vi "CSMOMgr-Get CSMO.vi"(6 "GenError?(T)":bool=TRUE, 8 "Error in":errorcluster caption="Error in (no error)", 10 "Queue Name":string, 11 "CSMOMgr":T3) -> (0 "Error out":errorcluster, 1 "values":T1={"Requested Name"="", "Module Name"="", "Mode"=enum."Stand Alone", "Queue"=refnum, "CSM-Data"=refnum, "User Event"=refnum, "Status Change Event"=refnum, "Allowed Messages"=[], "Mode-Data"=refnum, "Group Name"="", "Exit Event"=refnum}, 2 "found":bool, 3 "CSMOMgr out":T3)   [LabVIEW 2020, in "Communicable State Machine.lvlib"]
uses:
  Communicable State Machine.lvlib
  Def-CSMOMgr.ctl
  _CSMObj.ctl
  Priority Queue.lvclass
  _CSM_MODE.ctl
  _CSMObj-Data.ctl
  _CSM Status Change Event Data.ctl
  _CSMObj-ModeData.ctl
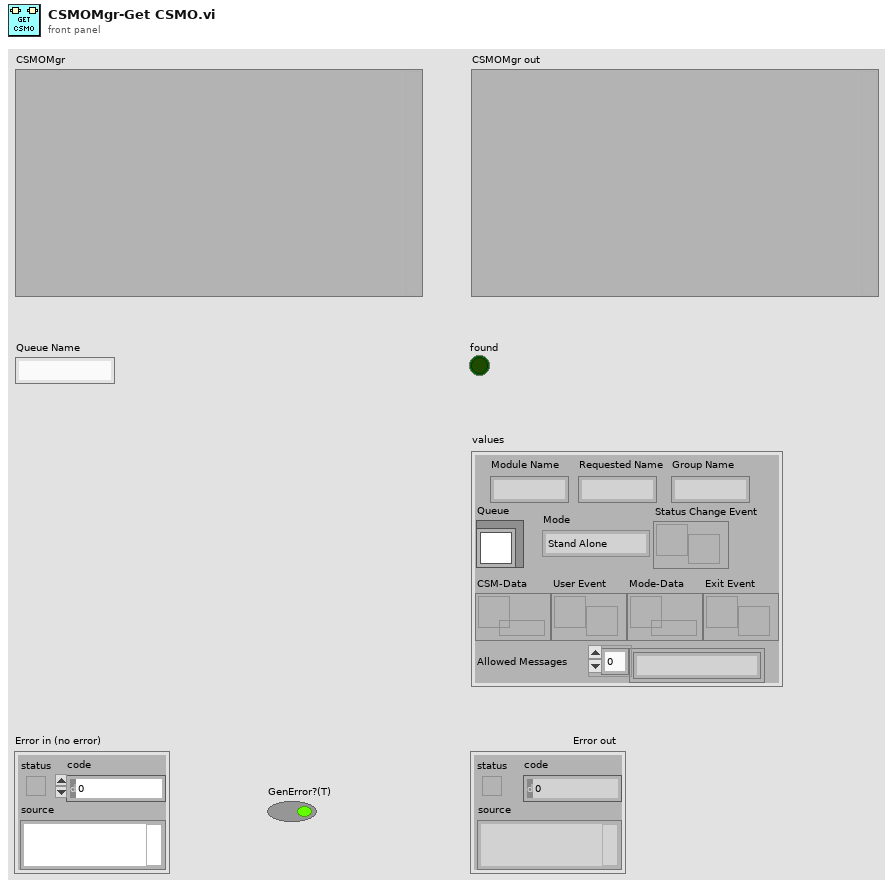
[diagram p1: front panel]
types:
  T1 = typedef "Communicable State Machine.lvlib/_CSMObj.ctl" = cluster{"Requested Name":string, "Module Name":string, "Mode":T2, "Queue":refnum<class "Priority Queue.lvclass">, "CSM-Data":refnum<data-value>, "User Event":refnum<user-event>, "Status Change Event":refnum<user-event>, "Allowed Messages":string[], "Mode-Data":refnum<data-value>, "Group Name":string, "Exit Event":refnum<user-event>}
  T2 = typedef "Communicable State Machine.lvlib/_CSM_MODE.ctl" = enum16{"Not Exist", "Stand Alone", "CSM", "Worker Agent", "Worker", "Chain", "Chain Node"}
  T3 = typedef "Communicable State Machine.lvlib/Def-CSMOMgr.ctl" = variant
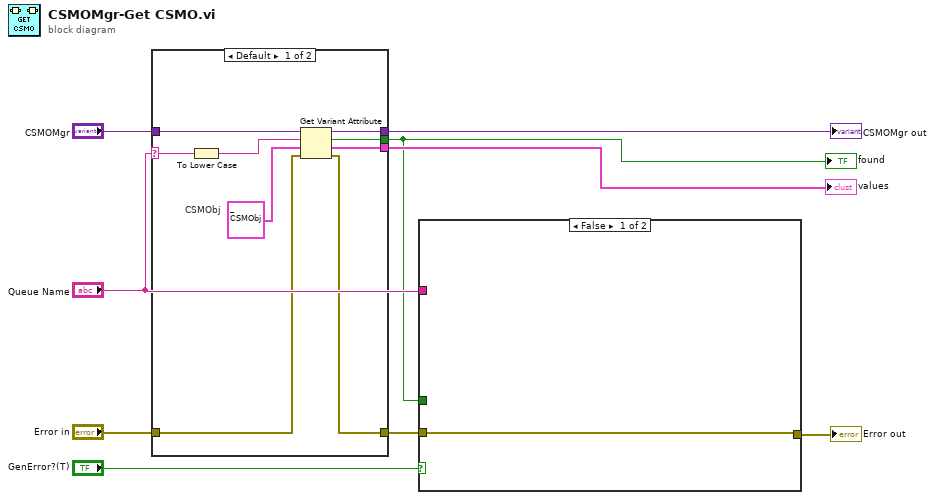
[diagram p0: block diagram]
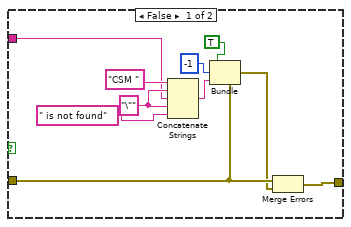
[diagram p4: hidden frame]
diagram:
  n1 = case shown="Default" "Queue Name" {
    selector: "Queue Name" -> [w12 _]
    tunnel: "CSMOMgr" -> [w18 w20]
    tunnel: [w17 w20] -> w8
    tunnel: "Error in" -> [w16 w19]
    tunnel: [w14 w19] -> w6
    tunnel: [w13 _] -> w4
    tunnel: [w11 _] -> w2
    frame Default {
      w15 = T1 {"Requested Name"="", "Module Name"="", "Mode"=enum."Not Exist", "Queue"=refnum, "CSM-Data"=refnum, "User Event"=refnum, "Status Change Event"=refnum, "Allowed Messages"=[], "Mode-Data"=refnum, "Group Name"="", "Exit Event"=refnum}  # CSMObj
      n2 = To Lower Case(string=w12) -> (all lower case string=w10:string)
      n3 = Get Variant Attribute(Variant=w18, name=w10, default value (empty Variant)=w15, error in=w16) -> (duplicate Variant=w17:variant, found=w11:bool, value=w13:T1, error out=w14:errorcluster)
    }
    frame "" {
    }
  }
  "CSMOMgr out" <- w8
  "values" <- w4
  "found" <- w2
  n4 = case shown="False" "GenError?(T)" {
    tunnel: w6 -> [w21 w25]
    tunnel: [w21 w24] -> w5
    tunnel: "Queue Name" -> [_ w23]
    tunnel: w2 -> [_ w22]
    frame False {
    }
    frame True {
      n5 = case shown="True" w22 {
        tunnel: w25 -> [w28 w36]
        tunnel: [w27 w36] -> w24
        tunnel: w23 -> [w29 _]
        frame False {
          w33 = "\"" ("string")
          n6 = Concatenate Strings("CSM " ("String to Prepend to source (\"\")"), w33, w29, w33, " is not found" ("string")) -> (w34:string)
          n7 = Bundle(cluster=w28, "status"=TRUE, "code"=-1, "source"=w34) -> (w26:errorcluster)
          n8 = Merge Errors(w28, w26) -> (w27:errorcluster)
        }
        frame True {
        }
      }
    }
  }
  "Error out" <- w5
